vi "test Scheduled Tx Encode Parameters into Words for Labels in a Channel.vi"(8 "error in":errorcluster, 11 "TestCase in":refnum<class "Engine.lvclass">) -> (0 "error out":errorcluster, 3 "TestCase out":refnum<class "Engine.lvclass">)   [LabVIEW 2024, in "Engine.lvclass"]
uses:
  Engine.lvclass
  Shared/RT Label Settings.ctl
  Shared/Label.ctl
  Shared/RT Parameters.ctl
  Shared/Parameter Definition.ctl
  <vilib>/NI/NI VeriStand Encoding and Decoding/Encoding.ctl
  <vilib>/NI VeriStand/Custom Device API/Custom Device Item Ref.ctl
  Shared/Transfer Type.ctl
  <vilib>/NI VeriStand/Custom Device API/Data Reference.ctl
  <vilib>/addons/_JKI Toolkits/VI Tester/TestCase.llb/TestCase.lvclass
  <vilib>/NI VeriStand/Custom Device API/Custom Device API.lvlib
  <vilib>/NI/NI VeriStand Encoding and Decoding/Encoding and Decoding.lvlib
  Engine/Implementation/Tx Scheduled Labels Execution Unit/Tx Scheduled Labels Execution Unit.lvclass
  C:/Program Files/National Instruments/LabVIEW 2024/vi.lib/addons/_JKI Toolkits/VI Tester/TestCase.llb/TestCase.lvclass
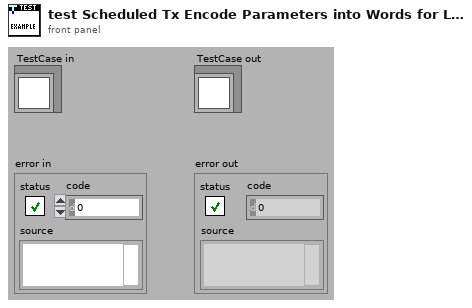
[diagram p1: front panel]
types:
  T1 = typedef "RT Label Settings.ctl" = cluster{"Name":string, "xmlName":string, "label":T2, "transfer period":u32, "SDI_Enabled":bool, "SDI":u8, "parameter driver data":T3, "transfer type":T7, "has timestamp?":bool, "Label Disable/Trigger Channel Reference":T6, "Message Handle":u64, "Initialized?":bool, "Word Initial Raw Value":u32, "Label Timestamp Channel Data Reference":T8, "disabled":bool, "modified":bool}
  T2 = typedef "Label.ctl" = u8
  T3 = typedef "RT Parameters.ctl" = cluster{"parameter definitions":T4[], "Tx parameter refs":T6[]}
  T4 = typedef "Parameter Definition.ctl" = cluster{"start index":i32, "size":i32, "encoding":T5, "signed":bool, "scale multiplier":dbl, "scale offset":dbl, "default value":dbl}
  T5 = typedef "Encoding and Decoding.lvlib/Encoding.ctl" = enum16{"BNR", "BCD", "Discrete"}
  T6 = typedef "Custom Device API.lvlib/Custom Device Item Ref.ctl" = u64
  T7 = typedef "Transfer Type.ctl" = enum16{"Scheduled", "Acyclic", "Block", "Strobe"}
  T8 = typedef "Custom Device API.lvlib/Data Reference.ctl" = i32
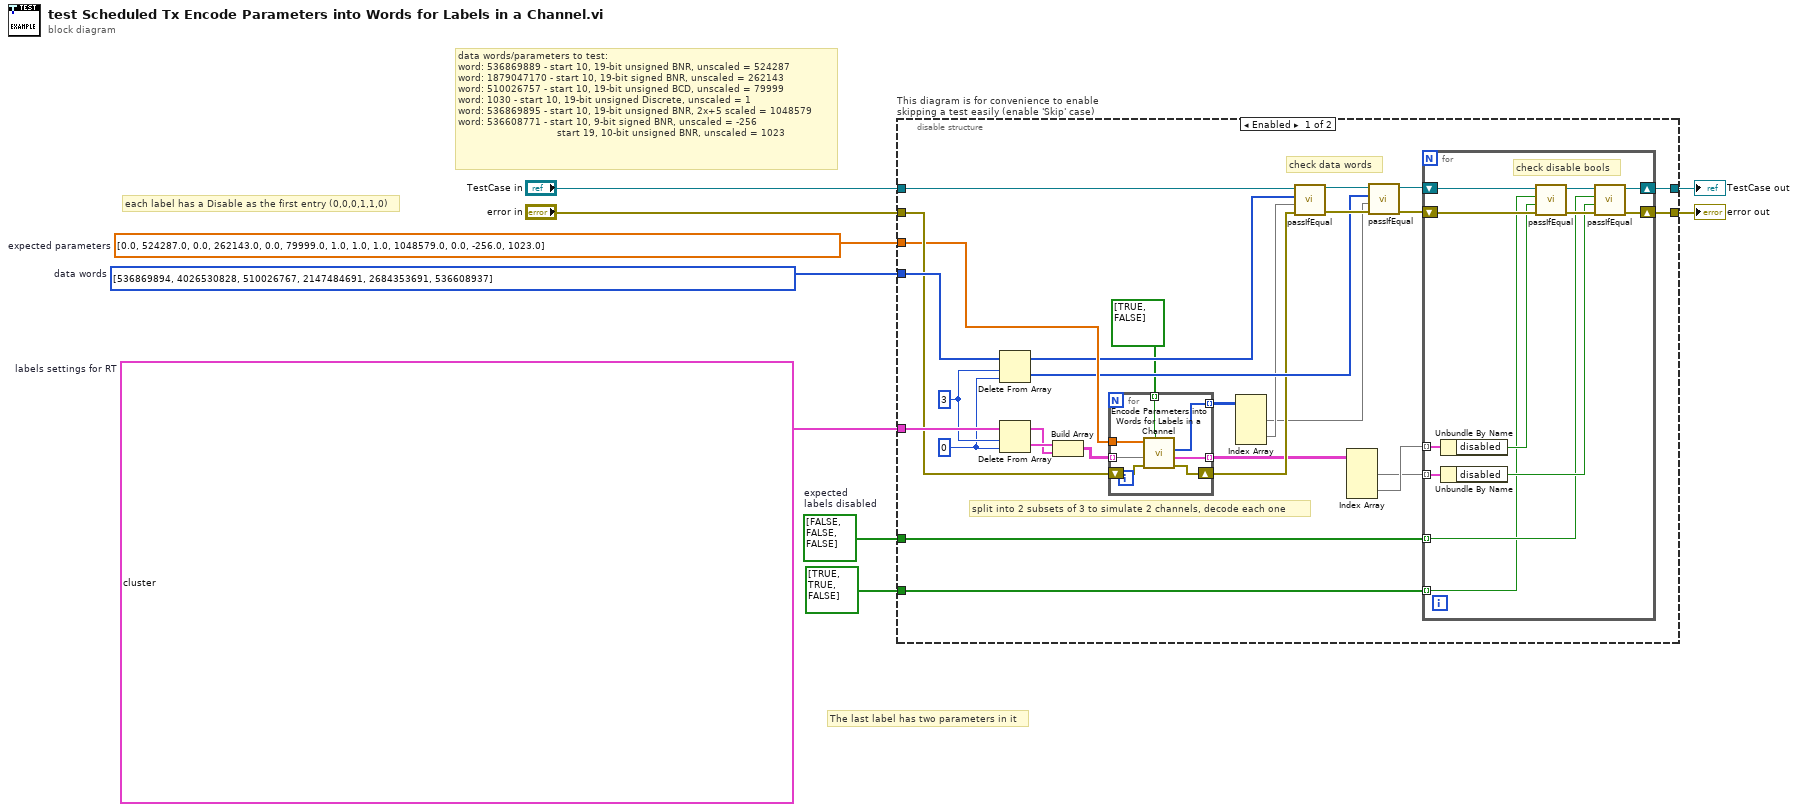
[diagram p0: block diagram]
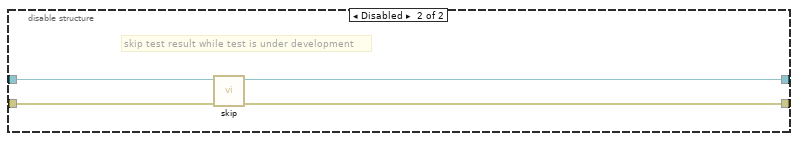
[diagram p2: hidden frame]
diagram:
  w2 = bool[] [FALSE, FALSE, FALSE]  # expected labels disabled
  w4 = dbl[] [0.0, 524287.0, 0.0, 262143.0, 0.0, 79999.0, 1.0, 1.0, 1.0, 1048579.0, 0.0, -256.0, 1023.0]  # expected parameters
  w5 = T1[] [{"Name"="", "xmlName"="", "label"=6, "transfer period"=10, "SDI_Enabled"=FALSE, "SDI"=0, "parameter driver data"={"parameter definitions"=[{"start index"=10, "size"=19, "encoding"=enum."BNR", "signed"=FALSE, "scale multiplier"=1.0, "scale offset"=0.0, "default value"=0.0}], "Tx parameter refs"=[]}, "transfer type"=enum."Scheduled", "has timestamp?"=FALSE, "Label Disable/Trigger Channel Reference"=0, "Message Handle"=0, "Initialized?"=FALSE, "Word Initial Raw Value"=0, "Label Timestamp Channel Data Reference"=0, "disabled"=FALSE, "modified"=FALSE}, {"Name"="", "xmlName"="", "label"=12, "transfer period"=10, "SDI_Enabled"=FALSE, "SDI"=0, "parameter driver data"={"parameter definitions"=[{"start index"=10, "size"=19, "encoding"=enum."BNR", "signed"=TRUE, "scale multiplier"=1.0, "scale offset"=0.0, "default value"=0.0}], "Tx parameter refs"=[]}, "transfer type"=enum."Scheduled", "has timestamp?"=FALSE, "Label Disable/Trigger Channel Reference"=0, "Message Handle"=0, "Initialized?"=FALSE, "Word Initial Raw Value"=0, "Label Timestamp Channel Data Reference"=0, "disabled"=FALSE, "modified"=FALSE}, {"Name"="", "xmlName"="", "label"=15, "transfer period"=10, "SDI_Enabled"=FALSE, "SDI"=0, "parameter driver data"={"parameter definitions"=[{"start index"=10, "size"=19, "encoding"=enum."BCD", "signed"=FALSE, "scale multiplier"=1.0, "scale offset"=0.0, "default value"=0.0}], "Tx parameter refs"=[]}, "transfer type"=enum."Scheduled", "has timestamp?"=FALSE, "Label Disable/Trigger Channel Reference"=0, "Message Handle"=0, "Initialized?"=FALSE, "Word Initial Raw Value"=0, "Label Timestamp Channel Data Reference"=0, "disabled"=FALSE, "modified"=FALSE}, {"Name"="", "xmlName"="", "label"=19, "transfer period"=10, "SDI_Enabled"=FALSE, "SDI"=0, "parameter driver data"={"parameter definitions"=[{"start index"=10, "size"=19, "encoding"=enum."Discrete", "signed"=FALSE, "scale multiplier"=1.0, "scale offset"=0.0, "default value"=0.0}], "Tx parameter refs"=[]}, "transfer type"=enum."Scheduled", "has timestamp?"=FALSE, "Label Disable/Trigger Channel Reference"=0, "Message Handle"=0, "Initialized?"=FALSE, "Word Initial Raw Value"=0, "Label Timestamp Channel Data Reference"=0, "disabled"=FALSE, "modified"=FALSE}, {"Name"="", "xmlName"="", "label"=155, "transfer period"=10, "SDI_Enabled"=FALSE, "SDI"=0, "parameter driver data"={"parameter definitions"=[{"start index"=10, "size"=19, "encoding"=enum."BNR", "signed"=FALSE, "scale multiplier"=2.0, "scale offset"=5.0, "default value"=0.0}], "Tx parameter refs"=[]}, "transfer type"=enum."Scheduled", "has timestamp?"=FALSE, "Label Disable/Trigger Channel Reference"=0, "Message Handle"=0, "Initialized?"=FALSE, "Word Initial Raw Value"=0, "Label Timestamp Channel Data Reference"=0, "disabled"=FALSE, "modified"=FALSE}, {"Name"="", "xmlName"="", "label"=169, "transfer period"=10, "SDI_Enabled"=FALSE, "SDI"=0, "parameter driver data"={"parameter definitions"=[{"start index"=10, "size"=9, "encoding"=enum."BNR", "signed"=TRUE, "scale multiplier"=1.0, "scale offset"=0.0, "default value"=0.0}, {"start index"=19, "size"=10, "encoding"=enum."BNR", "signed"=FALSE, "scale multiplier"=1.0, "scale offset"=0.0, "default value"=0.0}], "Tx parameter refs"=[]}, "transfer type"=enum."Scheduled", "has timestamp?"=FALSE, "Label Disable/Trigger Channel Reference"=0, "Message Handle"=0, "Initialized?"=FALSE, "Word Initial Raw Value"=0, "Label Timestamp Channel Data Reference"=0, "disabled"=FALSE, "modified"=FALSE}]  # labels settings for RT
  w6 = u32[] [536869894, 4026530828, 510026767, 2147484691, 2684353691, 536608937]  # data words
  # "each label has a Disable as the first entry (0,0,0,1,1,0)"
  # "The last label has two parameters in it"
  # "for visibility, irrelevant label settings are minimized in this constant"
  # "data words/parameters to test:\nword: 536869889 - start 10, 19-bit unsigned BNR, unscaled = 524287\nword: 1879047170 - start 10, 19-bit signed BNR, unscaled = 262143\nword: 510026757 - start 10, 19-bit unsigned BCD, unscaled = 79999\nword: 1030 - start 10, 19-bit unsigned Discrete, unscaled = 1\nword: 536869895 - start 10, 19-bit unsigned BNR, 2x+5 scaled = 1048579 \nword: 536608771 - start 10, 9-bit signed BNR, unscaled = -256\n                                 start 19, 10-bit unsigned BNR, unscaled = 1023"
  n1 = disable-structure "This diagram is for convenience to enable skipping a test easily (enable 'Skip' case)" shown="Enabled" {
    disable-tunnel: "TestCase in" -> [w35 w60]
    disable-tunnel: [w30 w58] -> w3
    disable-tunnel: [w29 w59] -> w8
    disable-tunnel: "error in" -> [w32 w57]
    disable-tunnel: w6 -> [w36 _]
    disable-tunnel: w5 -> [w37 _]
    disable-tunnel: w4 -> [w31 _]
    disable-tunnel: w2 -> [w28 _]
    disable-tunnel: bool[] [TRUE, TRUE, FALSE] -> [w27 _]
    frame Enabled {
      w33 = 0 ("index")
      w34 = 3 ("length")
      # "check data words"
      # "split into 2 subsets of 3 to simulate 2 channels, decode each one"
      n2 = Delete From Array(array=w36, length=w34, index=w33) -> (deleted portion=w22:u32[], array with subset deleted=w21:u32[])
      n3 = Delete From Array(array=w37, length=w34, index=w33) -> (deleted portion=w20:T1[], array with subset deleted=w19:T1[])
      n4 = Build Array(w20, w19) -> (w18:T1[][])
      n5 = for {
        tunnel: w31 -> [w38]
        tunnel: w18 -> [w43] mode=indexing
        tunnel: bool[] [TRUE, FALSE] ("reset index") -> [w42] mode=indexing
        tunnel: [w40] -> w15 mode=indexing
        tunnel: [w39] -> w14 mode=indexing
        shift-right: [w41] -> w16
        shift-left: w32 -> [w44]
        n6 = call "Encode Parameters into Words for Labels in a Channel.vi"("reset index"=w42, "error in (no error)"=w44, "labels settings for RT in"=w43, "Parameter Values in"=w38) -> ("error out"=w41:errorcluster, "labels settings for RT out"=w40:T1[], "data words out"=w39:u32[])  [unwired: 5 in]
      }
      n7 = Index Array(array=w14) -> (element #1=w12:u32[], element #2=w13:u32[])  [unwired: 4 in]
      n8 = call-dynamic "passIfEqual.vi"("error in (no error)"=w16, "y"=w13, "x"=w21, "TestCase in"=w35) -> ("error out"=w23:errorcluster, "TestCase out"=w24:refnum<class "Engine.lvclass">)  [unwired: 6 in]
      n9 = Index Array(array=w15) -> (element #1=w10:T1[], element #2=w11:T1[])  [unwired: 4 in]
      n10 = call-dynamic "passIfEqual.vi"("error in (no error)"=w23, "y"=w12, "x"=w22, "TestCase in"=w24) -> ("error out"=w26:errorcluster, "TestCase out"=w25:refnum<class "Engine.lvclass">)  [unwired: 6 in]
      n11 = for {
        shift-right: [w49] -> w30
        shift-left: w25 -> [w56]
        shift-right: [w48] -> w29
        shift-left: w26 -> [w55]
        tunnel: w10 -> [w53] mode=indexing
        tunnel: w11 -> [w54] mode=indexing
        tunnel: w28 -> [w46] mode=indexing
        tunnel: w27 -> [w45] mode=indexing
        # "check disable bools"
        n12 = Unbundle By Name(w54) -> ("disabled"=w52:bool)
        n13 = Unbundle By Name(w53) -> ("disabled"=w47:bool)
        n14 = call-dynamic "passIfEqual.vi"("error in (no error)"=w55, "y"=w52, "x"=w45, "TestCase in"=w56) -> ("error out"=w50:errorcluster, "TestCase out"=w51:refnum<class "Engine.lvclass">)  [unwired: 6 in]
        n15 = call-dynamic "passIfEqual.vi"("error in (no error)"=w50, "y"=w47, "x"=w46, "TestCase in"=w51) -> ("error out"=w48:errorcluster, "TestCase out"=w49:refnum<class "Engine.lvclass">)  [unwired: 6 in]
      }
    }
    frame Disabled {
      # "skip test result while test is under development"
      n16 = call <vilib>:"skip.vi"("error in (no error)"=w57, "TestCase in"=w60) -> ("error out"=w59:errorcluster, "TestCase out"=w58:refnum<class "Engine.lvclass">)  [unwired: 8 in]
    }
  }
  "error out" <- w8
  "TestCase out" <- w3
